vi "Get Public API.vi"(8 "error in (no error)":errorcluster, 11 "Instrument.VoltageSource in":refnum<class "Instrument.VoltageSource.lvclass">) -> (0 "error out":errorcluster, 2 "Commands":string[](array[string]), 3 "Instrument.VoltageSource out":refnum<class "Instrument.VoltageSource.lvclass">)   [LabVIEW 2016, in "Instrument.VoltageSource.lvclass"]
uses:
  Instrument.VoltageSource.lvclass
  <userlib>/LevyLab/Levylab Instruments/Instrument Types/VSource/Instrument.VSource.lvclass
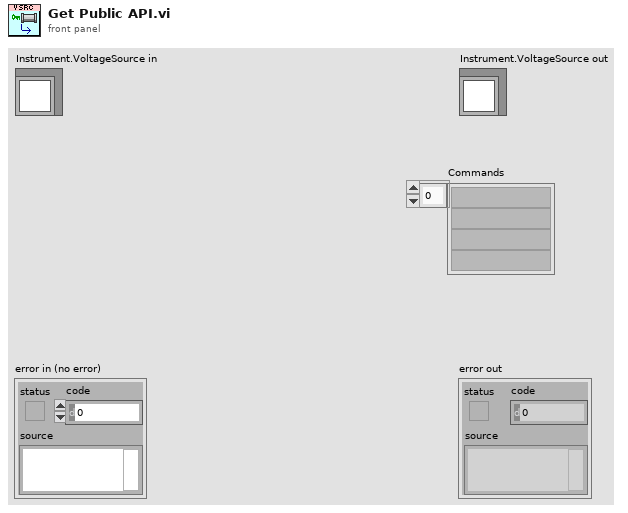
[diagram p1: front panel]
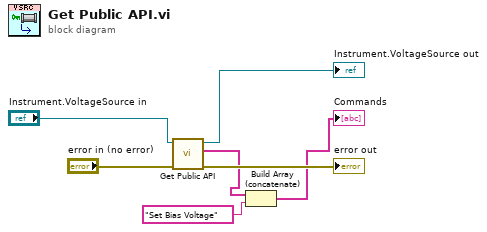
[diagram p0: block diagram]
diagram:
  n1 = call-parent "Get Public API.vi"("error in (no error)"="error in (no error)", "Instrument in"="Instrument.VoltageSource in") -> ("error out"=→"error out":errorcluster, "Commands"=w3:string[], "Instrument out"=→"Instrument.VoltageSource out":refnum<class "Instrument.VoltageSource.lvclass">)  [unwired: 7 in]
  n2 = Build Array (concatenate)(w3, "Set Bias Voltage") -> (→"Commands":string[])
